vi "ziGetValueAsPoll.vi"(3 "error in":errorcluster, 4 "Path":string, 5 "Handle in":T1 {"Handle" format="0x%08x"; "Conn" format="0x%08x"}) -> (0 "error out":errorcluster, 2 "Handle out":T1 {"Handle" format="0x%08x"; "Conn" format="0x%08x"})   [LabVIEW 2009, in "Zurich Instruments LabOne.lvlib"]
doc: "Use this vi to receive the value of one or more nodes as events using ziPollDataEx, even when the node is not subscribed or no value change has occured."
uses:
  <instrlib>/Zurich Instruments LabOne/Zurich Instruments LabOne.lvlib
  <instrlib>/Zurich Instruments LabOne/Public/ziTypeHandle.ctl
  <instrlib>/Zurich Instruments LabOne/Private/ziLV32.dll
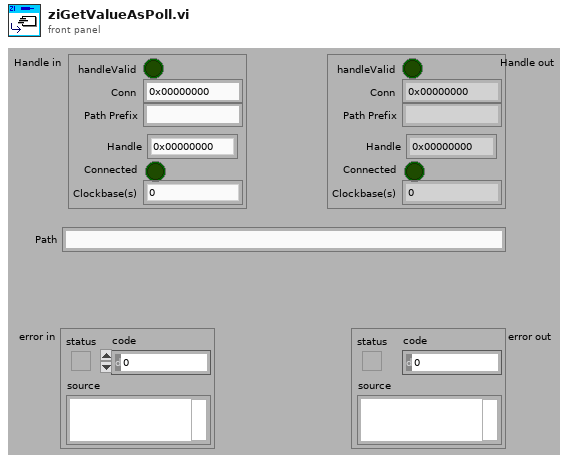
[diagram p1: front panel]
types:
  T1 = typedef "Zurich Instruments LabOne.lvlib/ziTypeHandle.ctl" = cluster{"handleValid":bool, "Conn":u64, "Path Prefix":string, "Handle":u64, "Connected":bool, "Clockbase(s)":dbl}
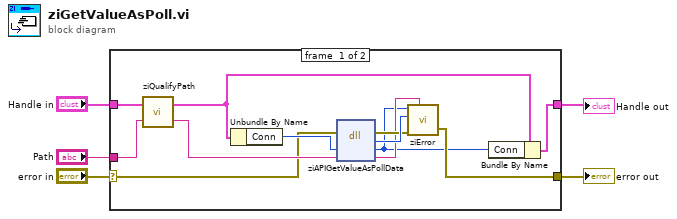
[diagram p0: block diagram]
diagram:
  n1 = case shown="No Error" "error in" {
    selector: "error in" -> [w7 w18]
    tunnel: [w14 w18] -> w5
    tunnel: [w13 w19] -> w4
    tunnel: "Handle in" -> [w12 w19]
    tunnel: "Path" -> [w10 _]
    frame #0 {
      n2 = call <instrlib>:"ziQualifyPath.vi"("Path In"=w10, "Handle In"=w12) -> ("Path Out"=w9:string, "Handle Out"=w11:T1)
      n3 = Unbundle By Name(w11) -> ("Conn"=w17:u64)
      n4 = dll-call lib="C:/Program Files (x86)/National Instruments/LabVIEW 2009/instr.lib/Zurich Instruments LabOne/Private/ziLV*.*" fn="ziAPIGetValueAsPollData" ("ZestSC1.dll:ZestSC1CountCards")(error in=w7, "Conn"=w17, "Path"=w9) -> (error out=w15:errorcluster, "return type"=w16:u32, "Conn"=w6:u64, "Path"=w8:string)  [unwired: 2 in, 1 out]
      n5 = call <instrlib>:"ziError.vi"("Conn"=w6, "ziErrorCode"=w16, "Error In"=w15, "Annotation"=w8) -> ("Error Out"=w14:errorcluster)  [unwired: 1 in, 1 out]
      n6 = Bundle By Name(cluster=w11, "Conn"=w6) -> (w13:T1)
    }
    frame #1 {
    }
  }
  "Handle out" <- w4
  "error out" <- w5
